vi "Hot Goal Recognition.vi"() -> (0 "Right Goal Hot?":bool, 1 "Left Goal hot?":bool)   [LabVIEW 2013]
uses:
  <vilib>/Rock Robotics/WPI/Camera/WPI_CameraSettings Read MJPG.ctl
  <vilib>/Rock Robotics/WPI/Camera/WPI_CameraImageSize.ctl
  <vilib>/vision/NI_Vision_Development_Module.lvlib
panel:
  out "ERROR":bool
  out "Image":T1(plugin-control)
  out "error out":errorcluster
  in  "Camera IP":string="10.9.0.11"
  out "Bandwidth (Mbps)":dbl
  in  "Camera Settings":T2={"fps"=30, "compression"=30, "Image Size"=enum."320x240"}
  # "do not change resolution!!!! (320x240)"
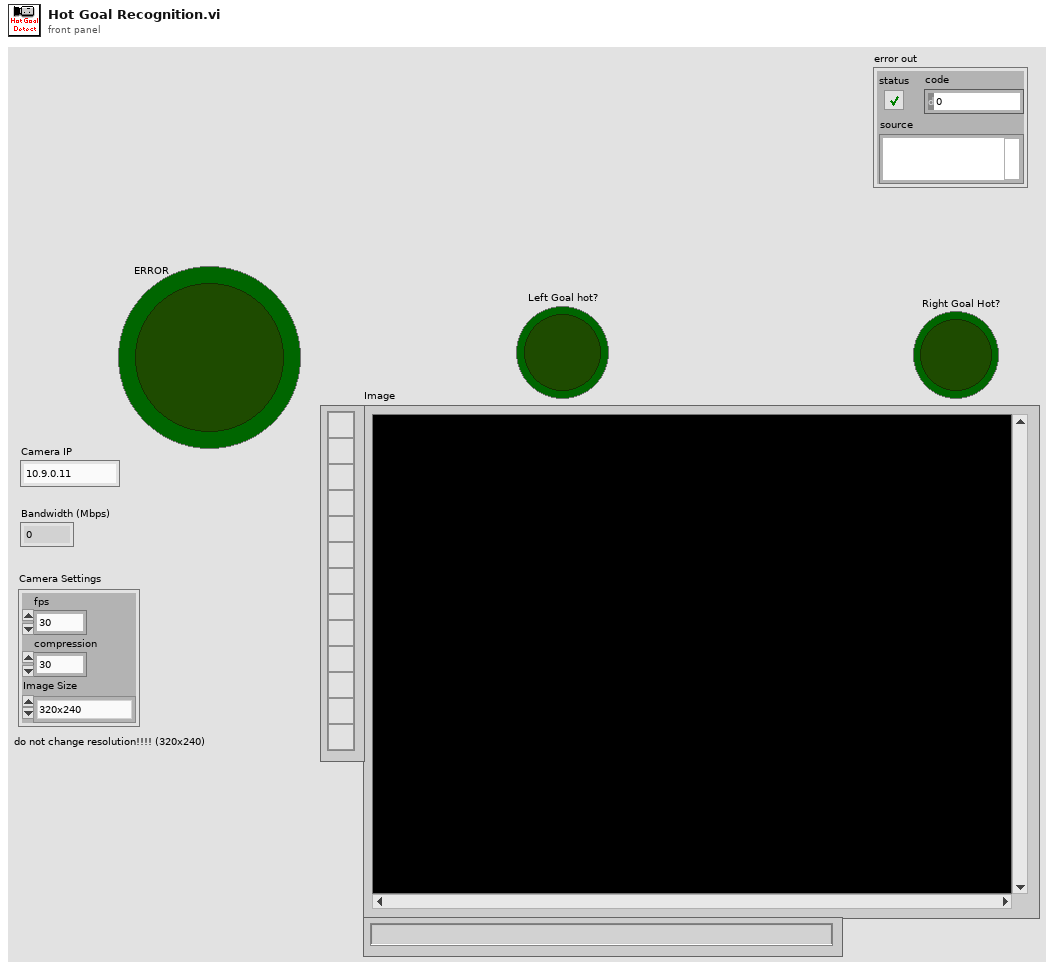
[diagram p1: front panel]
types:
  T1 = typedef "IMAQ Image.ctl" = refnum<image>
  T2 = typedef "WPI_CameraSettings Read MJPG.ctl" = cluster{"fps":i32, "compression":i32, "Image Size":T3}
  T3 = typedef "WPI_CameraImageSize.ctl" = enum16{"640x480", "320x240", "160x120"}
  T4 = typedef "Image Type" = u32
  T5 = enum32{"AutoM", "Close", "Dilate", "Erode", "Gradient", "Gradient in", "Gradient out", "HitMiss", "Open", "PClose", "POpen", "Thick", "Thin"}
  T6 = typedef "Particle Parameters" = i32
  T7 = cluster{"Particle Measurements (Pixels)[0]":dbl, "Particle Measurements (Pixels)[1]":dbl}
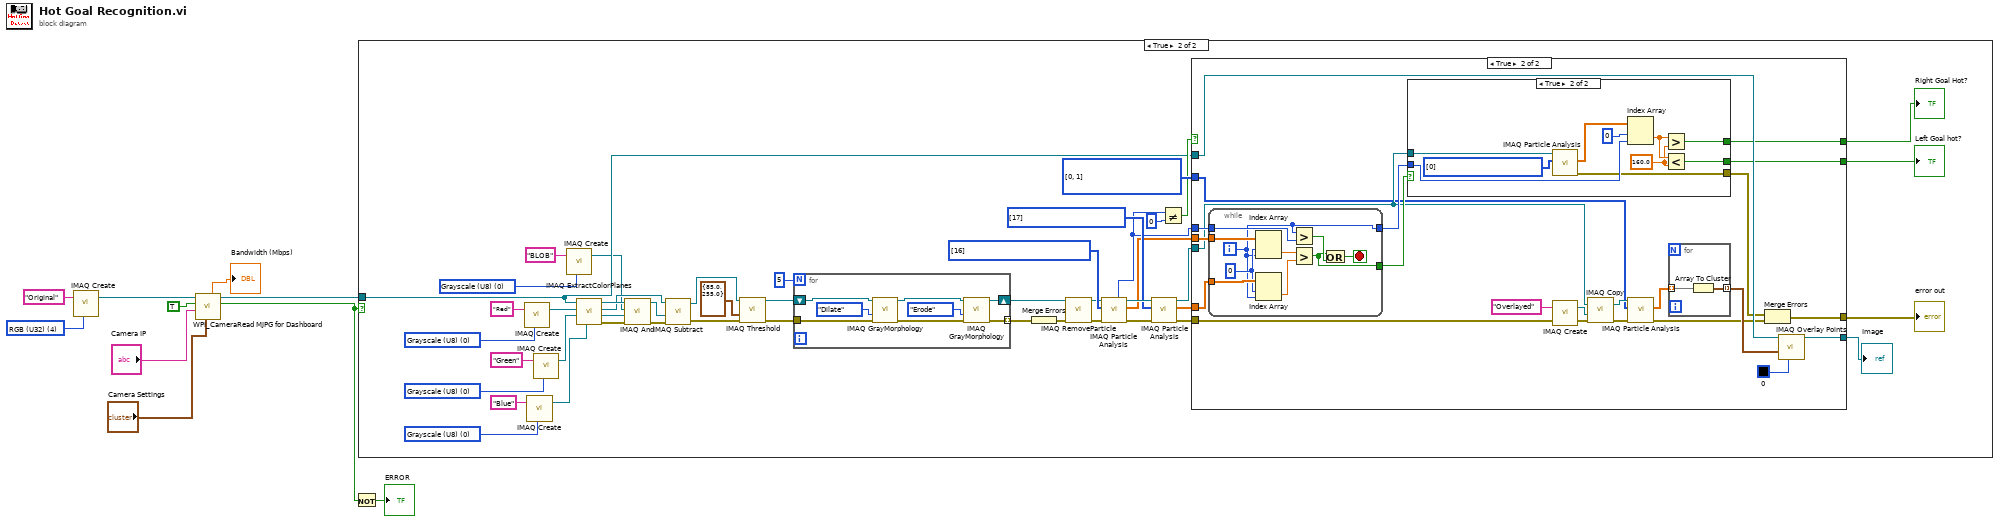
[diagram p0: block diagram]
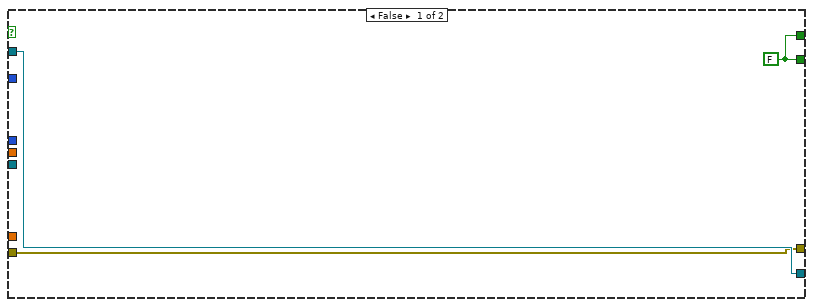
[diagram p3: hidden frame]
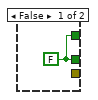
[diagram p4: hidden frame]
diagram:
  w1 = T4 4 items=["Grayscale (U8)", "Grayscale (I16)", "Grayscale (SGL)", "Complex (CSG)", "RGB (U32)", "HSL (U32)", "RGB (U64)", "Grayscale (U16)"] ("Image Type")
  n1 = call "IMAQ Create"("Image Name"="Original", "Image Type"=w1) -> ("New Image"=w9:T1)  [unwired: 3 in, 1 out]
  n2 = call <vilib>:"WPI_CameraRead MJPG for Dashboard.vi"("Camera Settings"="Camera Settings", "Camera IP"="Camera IP", "Enable"=TRUE, "Refnum in"=w9) -> ("Active"=w6:bool, "Refnum out"=w7:T1, "Bandwidth (Mbps)"=→"Bandwidth (Mbps)":dbl)  [unwired: 4 in, 1 out]
  n3 = Not(x=w6) -> (.not. x?=→"ERROR":bool)
  n4 = case shown="True" w6 {
    tunnel: w7 -> [_ w25]
    frame False {
    }
    frame True {
      w30 = T6[] [0, 1] items=["Center of Mass X", "Center of Mass Y", "First Pixel X", "First Pixel Y", "Bounding Rect Left", "Bounding Rect Top", "Bounding Rect Right", "Bounding Rect Bottom", "Max Feret Diameter Start X", "Max Feret Diameter Start Y", "Max Feret Diameter End X", "Max Feret Diameter End Y", "Max Horiz. Segment Length Left", "Max Horiz. Segment Length Right", "Max Horiz. Segment Length Row", "-", "Bounding Rect Width", "Bounding Rect Height", "Bounding Rect Diagonal", "Perimeter", "Convex Hull Perimeter", "Holes' Perimeter", "Max Feret Diameter", "Equivalent Ellipse Major Axis", "Equivalent Ellipse Minor Axis", "Equivalent Ellipse Minor Axis (Feret)", "Equivalent Rect Long Side", "Equivalent Rect Short Side", "Equivalent Rect Diagonal", "Equivalent Rect Short Side (Feret)", "Average Horiz. Segment Length", "Average Vert. Segment Length", "Hydraulic Radius", "Waddel Disk Diameter", "-", "Area", "Holes' Area", "Particle & Holes' Area", "Convex Hull Area", "Image Area", "-", "Number of Holes", "Number of Horiz. Segments", "Number of Vert. Segments", "-", "Orientation", "Max Feret Diameter Orientation", "-", "% Area/Image Area", "% Area/(Particle & Holes' Area)", "Ratio of Equivalent Ellipse Axes", "Ratio of Equivalent Rect Sides", "-", "Elongation Factor", "Compactness Factor", "Heywood Circularity Factor", "Type Factor", "-", "Sum X", "Sum Y", "Sum XX", "Sum XY", "Sum YY", "Sum XXX", "Sum XXY", "Sum XYY", "Sum YYY", "-", "Moment of Inertia XX", "Moment of Inertia XY", "Moment of Inertia YY", "Moment of Inertia XXX", "Moment of Inertia XXY", "Moment of Inertia XYY", "Moment of Inertia YYY", "Norm. Moment of Inertia XX", "Norm. Moment of Inertia XY", "Norm. Moment of Inertia YY", "Norm. Moment of Inertia XXX", "Norm. Moment of Inertia XXY", "Norm. Moment of Inertia XYY", "Norm. Moment of Inertia YYY", "Hu Moment 1", "Hu Moment 2", "Hu Moment 3", "Hu Moment 4", "Hu Moment 5", "Hu Moment 6", "Hu Moment 7"] ("Pixel Measurements")
      w42 = T4 0 items=["Grayscale (U8)", "Grayscale (I16)", "Grayscale (SGL)", "Complex (CSG)", "RGB (U32)", "HSL (U32)", "RGB (U64)", "Grayscale (U16)"] ("Image Type")
      w45 = T4 0 items=["Grayscale (U8)", "Grayscale (I16)", "Grayscale (SGL)", "Complex (CSG)", "RGB (U32)", "HSL (U32)", "RGB (U64)", "Grayscale (U16)"] ("Image Type")
      w47 = T4 0 items=["Grayscale (U8)", "Grayscale (I16)", "Grayscale (SGL)", "Complex (CSG)", "RGB (U32)", "HSL (U32)", "RGB (U64)", "Grayscale (U16)"] ("Image Type")
      w52 = T6[] [17] items=["Center of Mass X", "Center of Mass Y", "First Pixel X", "First Pixel Y", "Bounding Rect Left", "Bounding Rect Top", "Bounding Rect Right", "Bounding Rect Bottom", "Max Feret Diameter Start X", "Max Feret Diameter Start Y", "Max Feret Diameter End X", "Max Feret Diameter End Y", "Max Horiz. Segment Length Left", "Max Horiz. Segment Length Right", "Max Horiz. Segment Length Row", "-", "Bounding Rect Width", "Bounding Rect Height", "Bounding Rect Diagonal", "Perimeter", "Convex Hull Perimeter", "Holes' Perimeter", "Max Feret Diameter", "Equivalent Ellipse Major Axis", "Equivalent Ellipse Minor Axis", "Equivalent Ellipse Minor Axis (Feret)", "Equivalent Rect Long Side", "Equivalent Rect Short Side", "Equivalent Rect Diagonal", "Equivalent Rect Short Side (Feret)", "Average Horiz. Segment Length", "Average Vert. Segment Length", "Hydraulic Radius", "Waddel Disk Diameter", "-", "Area", "Holes' Area", "Particle & Holes' Area", "Convex Hull Area", "Image Area", "-", "Number of Holes", "Number of Horiz. Segments", "Number of Vert. Segments", "-", "Orientation", "Max Feret Diameter Orientation", "-", "% Area/Image Area", "% Area/(Particle & Holes' Area)", "Ratio of Equivalent Ellipse Axes", "Ratio of Equivalent Rect Sides", "-", "Elongation Factor", "Compactness Factor", "Heywood Circularity Factor", "Type Factor", "-", "Sum X", "Sum Y", "Sum XX", "Sum XY", "Sum YY", "Sum XXX", "Sum XXY", "Sum XYY", "Sum YYY", "-", "Moment of Inertia XX", "Moment of Inertia XY", "Moment of Inertia YY", "Moment of Inertia XXX", "Moment of Inertia XXY", "Moment of Inertia XYY", "Moment of Inertia YYY", "Norm. Moment of Inertia XX", "Norm. Moment of Inertia XY", "Norm. Moment of Inertia YY", "Norm. Moment of Inertia XXX", "Norm. Moment of Inertia XXY", "Norm. Moment of Inertia XYY", "Norm. Moment of Inertia YYY", "Hu Moment 1", "Hu Moment 2", "Hu Moment 3", "Hu Moment 4", "Hu Moment 5", "Hu Moment 6", "Hu Moment 7"] ("Pixel Measurements")
      w54 = T6[] [16] items=["Center of Mass X", "Center of Mass Y", "First Pixel X", "First Pixel Y", "Bounding Rect Left", "Bounding Rect Top", "Bounding Rect Right", "Bounding Rect Bottom", "Max Feret Diameter Start X", "Max Feret Diameter Start Y", "Max Feret Diameter End X", "Max Feret Diameter End Y", "Max Horiz. Segment Length Left", "Max Horiz. Segment Length Right", "Max Horiz. Segment Length Row", "-", "Bounding Rect Width", "Bounding Rect Height", "Bounding Rect Diagonal", "Perimeter", "Convex Hull Perimeter", "Holes' Perimeter", "Max Feret Diameter", "Equivalent Ellipse Major Axis", "Equivalent Ellipse Minor Axis", "Equivalent Ellipse Minor Axis (Feret)", "Equivalent Rect Long Side", "Equivalent Rect Short Side", "Equivalent Rect Diagonal", "Equivalent Rect Short Side (Feret)", "Average Horiz. Segment Length", "Average Vert. Segment Length", "Hydraulic Radius", "Waddel Disk Diameter", "-", "Area", "Holes' Area", "Particle & Holes' Area", "Convex Hull Area", "Image Area", "-", "Number of Holes", "Number of Horiz. Segments", "Number of Vert. Segments", "-", "Orientation", "Max Feret Diameter Orientation", "-", "% Area/Image Area", "% Area/(Particle & Holes' Area)", "Ratio of Equivalent Ellipse Axes", "Ratio of Equivalent Rect Sides", "-", "Elongation Factor", "Compactness Factor", "Heywood Circularity Factor", "Type Factor", "-", "Sum X", "Sum Y", "Sum XX", "Sum XY", "Sum YY", "Sum XXX", "Sum XXY", "Sum XYY", "Sum YYY", "-", "Moment of Inertia XX", "Moment of Inertia XY", "Moment of Inertia YY", "Moment of Inertia XXX", "Moment of Inertia XXY", "Moment of Inertia XYY", "Moment of Inertia YYY", "Norm. Moment of Inertia XX", "Norm. Moment of Inertia XY", "Norm. Moment of Inertia YY", "Norm. Moment of Inertia XXX", "Norm. Moment of Inertia XXY", "Norm. Moment of Inertia XYY", "Norm. Moment of Inertia YYY", "Hu Moment 1", "Hu Moment 2", "Hu Moment 3", "Hu Moment 4", "Hu Moment 5", "Hu Moment 6", "Hu Moment 7"] ("Pixel Measurements")
      w55 = T4 0 items=["Grayscale (U8)", "Grayscale (I16)", "Grayscale (SGL)", "Complex (CSG)", "RGB (U32)", "HSL (U32)", "RGB (U64)", "Grayscale (U16)"] ("Image Type")
      n5 = call "IMAQ Create"("Image Name"="Red", "Image Type"=w47) -> ("New Image"=w48:T1)  [unwired: 3 in, 1 out]
      n6 = call "IMAQ Create"("Image Name"="Blue", "Image Type"=w42) -> ("New Image"=w41:T1)  [unwired: 3 in, 1 out]
      n7 = call "IMAQ Create"("Image Name"="Green", "Image Type"=w45) -> ("New Image"=w44:T1)  [unwired: 3 in, 1 out]
      n8 = call "IMAQ Create"("Image Name"="BLOB", "Image Type"=w55) -> ("New Image"=w12:T1)  [unwired: 3 in, 1 out]
      n9 = call "IMAQ ExtractColorPlanes"("Blue or Luma or Val or Inten Plane"=w41, "Green or Sat Plane"=w44, "Red or Hue Plane"=w48, "Image Src"=w25) -> ("error out"=w22:errorcluster, "Blue or Luma or Val or Inten Plane out"=w39:T1, "Green or Sat Plane out"=w38:T1, "Red or Hue Plane out"=w40:T1)  [unwired: 4 in]
      n10 = call "IMAQ And"("error in (no error)"=w22, "Image Src B"=w39, "Image Dst"=w12, "Image Src A"=w40) -> ("error out"=w19:errorcluster, "Image Dst Out"=w11:T1)  [unwired: 6 in]
      n11 = call "IMAQ Subtract"("Image Src A"=w38, "Image Src B"=w11, "error in (no error)"=w19) -> ("Image Dst Out"=w20:T1, "error out"=w18:errorcluster)  [unwired: 4 in]
      n12 = call "IMAQ Threshold"("error in (no error)"=w18, "Range"=cluster{"Lower value":sgl, "Upper value":sgl} {"Lower value"=85.0, "Upper value"=255.0}, "Image Src"=w20) -> ("error out"=w17:errorcluster, "Image Dst Out"=w21:T1)  [unwired: 7 in]
      n13 = for {
        N: 5 -> [_]
        shift-right: [w109] -> w13
        shift-left: w21 -> [w110]
        tunnel: w17 -> [w108]
        tunnel: [w106] -> w36 mode=indexing
        n14 = call "IMAQ GrayMorphology"("error in (no error)"=w108, "Operation"=T5."Dilate", "Image Src"=w110) -> ("error out"=w107:errorcluster, "Image Dst Out"=w111:T1)  [unwired: 7 in]
        n15 = call "IMAQ GrayMorphology"("error in (no error)"=w107, "Operation"=T5."Erode", "Image Src"=w111) -> ("error out"=w106:errorcluster, "Image Dst Out"=w109:T1)  [unwired: 7 in]
      }
      n16 = Merge Errors(w36) -> (w14:errorcluster)
      n17 = call "IMAQ RemoveParticle"("error in (no error)"=w14, "Image Src"=w13) -> ("error out"=w33:errorcluster, "Image Dst Out"=w34:T1)  [unwired: 8 in]
      n18 = call "IMAQ Particle Analysis"("error in (no error)"=w33, "Pixel Measurements"=w54, "Image"=w34) -> ("error out"=w35:errorcluster, "Particle Measurements (Pixels)"=w51:dbl[][], "Image Out (duplicate)"=w53:T1, "Number of Particles"=w29:i32)  [unwired: 3 in, 2 out]
      n19 = call "IMAQ Particle Analysis"("error in (no error)"=w35, "Pixel Measurements"=w52, "Image"=w53) -> ("error out"=w31:errorcluster, "Particle Measurements (Pixels)"=w50:dbl[][], "Image Out (duplicate)"=w32:T1)  [unwired: 3 in, 3 out]
      n20 = Not Equal?(x=w29, y=0) -> (x != y?=w27:bool)
      n21 = case shown="True" w27 {
        tunnel: w51 -> [_ w82]
        tunnel: w50 -> [_ w81]
        tunnel: w29 -> [_ w80]
        tunnel: w32 -> [_ w75]
        tunnel: w31 -> [w57 w74]
        tunnel: w30 -> [_ w70]
        tunnel: [w59 w66] -> w26
        tunnel: w25 -> [w59 w65]
        tunnel: [w58 w64] -> w24
        tunnel: [w58 w63] -> w23
        tunnel: [w57 w60] -> w15
        frame False {
          w58 = FALSE
        }
        frame True {
          n22 = while {
            tunnel: w82 -> [w104]
            tunnel: w81 -> [w105]
            tunnel: w80 -> [w98]
            tunnel: [w97] -> w78
            tunnel: [w96] -> w79
            i -> [w96]
            stop <- w99 stop-if-true
            w103 = 0 ("disabled index (row)")
            n23 = Index Array(array=w104, index (row)=w103, index (col)=w96) -> (element=w101:dbl)
            n24 = Index Array(array=w105, index (row)=w103, index (col)=w96) -> (element=w102:dbl)
            n25 = Greater?(x=w96, y=w98) -> (0:w100:bool)
            n26 = Greater?(x=w101, y=w102) -> (0:w97:bool)
            n27 = Or(x=w97, y=w100) -> (x .or. y?=w99:bool)
          }
          n28 = case shown="True" w78 {
            tunnel: w79 -> [_ w91]
            tunnel: w75 -> [_ w94]
            tunnel: [_ w90] -> w61
            tunnel: [w85 w87] -> w64
            tunnel: [w85 w86] -> w63
            frame False {
              w85 = FALSE
            }
            frame True {
              w88 = 160.0 ("y")
              w95 = T6[] [0] items=["Center of Mass X", "Center of Mass Y", "First Pixel X", "First Pixel Y", "Bounding Rect Left", "Bounding Rect Top", "Bounding Rect Right", "Bounding Rect Bottom", "Max Feret Diameter Start X", "Max Feret Diameter Start Y", "Max Feret Diameter End X", "Max Feret Diameter End Y", "Max Horiz. Segment Length Left", "Max Horiz. Segment Length Right", "Max Horiz. Segment Length Row", "-", "Bounding Rect Width", "Bounding Rect Height", "Bounding Rect Diagonal", "Perimeter", "Convex Hull Perimeter", "Holes' Perimeter", "Max Feret Diameter", "Equivalent Ellipse Major Axis", "Equivalent Ellipse Minor Axis", "Equivalent Ellipse Minor Axis (Feret)", "Equivalent Rect Long Side", "Equivalent Rect Short Side", "Equivalent Rect Diagonal", "Equivalent Rect Short Side (Feret)", "Average Horiz. Segment Length", "Average Vert. Segment Length", "Hydraulic Radius", "Waddel Disk Diameter", "-", "Area", "Holes' Area", "Particle & Holes' Area", "Convex Hull Area", "Image Area", "-", "Number of Holes", "Number of Horiz. Segments", "Number of Vert. Segments", "-", "Orientation", "Max Feret Diameter Orientation", "-", "% Area/Image Area", "% Area/(Particle & Holes' Area)", "Ratio of Equivalent Ellipse Axes", "Ratio of Equivalent Rect Sides", "-", "Elongation Factor", "Compactness Factor", "Heywood Circularity Factor", "Type Factor", "-", "Sum X", "Sum Y", "Sum XX", "Sum XY", "Sum YY", "Sum XXX", "Sum XXY", "Sum XYY", "Sum YYY", "-", "Moment of Inertia XX", "Moment of Inertia XY", "Moment of Inertia YY", "Moment of Inertia XXX", "Moment of Inertia XXY", "Moment of Inertia XYY", "Moment of Inertia YYY", "Norm. Moment of Inertia XX", "Norm. Moment of Inertia XY", "Norm. Moment of Inertia YY", "Norm. Moment of Inertia XXX", "Norm. Moment of Inertia XXY", "Norm. Moment of Inertia XYY", "Norm. Moment of Inertia YYY", "Hu Moment 1", "Hu Moment 2", "Hu Moment 3", "Hu Moment 4", "Hu Moment 5", "Hu Moment 6", "Hu Moment 7"] ("Pixel Measurements")
              n29 = call "IMAQ Particle Analysis"("Pixel Measurements"=w95, "Image"=w94) -> ("error out"=w90:errorcluster, "Particle Measurements (Pixels)"=w93:dbl[][])  [unwired: 4 in, 4 out]
              n30 = Index Array(array=w93, index (row)=0, index (col)=w91) -> (element=w89:dbl)
              n31 = Greater?(x=w89, y=w88) -> (0:w87:bool)
              n32 = Less?(x=w89, y=w88) -> (x < y?=w86:bool)
            }
          }
          n33 = call "IMAQ Create"("Image Name"="Overlayed", "error in (no error)"=w74) -> ("New Image"=w76:T1, "error out"=w73:errorcluster)  [unwired: 3 in]
          n34 = call "IMAQ Copy"("error in (no error)"=w73, "Image Dst"=w76, "Image Src"=w75) -> ("error out"=w72:errorcluster, "Image Dst Out"=w71:T1)  [unwired: 3 in]
          n35 = call "IMAQ Particle Analysis"("error in (no error)"=w72, "Pixel Measurements"=w70, "Image"=w71) -> ("error out"=w62:errorcluster, "Particle Measurements (Pixels)"=w67:dbl[][])  [unwired: 3 in, 4 out]
          n36 = for {
            tunnel: w67 -> [w84] mode=indexing
            tunnel: [w83] -> w68 mode=indexing
            n37 = Array To Cluster(array=w84) -> (cluster=w83:T7)
          }
          n38 = Merge Errors(w61, w62) -> (w60:errorcluster)
          n39 = call "IMAQ Overlay Points"("Color"=u32 0, "Array of Points"=w68, "Image"=w65) -> ("Image Out"=w66:T1)  [unwired: 7 in, 1 out]
        }
      }
      "error out" <- w15
      "Image" <- w26
      "Right Goal Hot?" <- w24
      "Left Goal hot?" <- w23
    }
  }
